vi "Get Command Field Width.vi"(8 "error in (no error)":errorcluster, 11 "RFFE Reg0Write Command in":refnum<class "RFFE Reg0Write Command.lvclass">) -> (0 "error out":errorcluster, 2 "Command Field Width":i32, 3 "RFFE Reg0Write Command out":refnum<class "RFFE Reg0Write Command.lvclass">)   [LabVIEW 2018, in "MIPI RFFE API.lvlib" / "RFFE Reg0Write Command.lvclass"]
uses:
  RFFE Reg0Write Command.lvclass
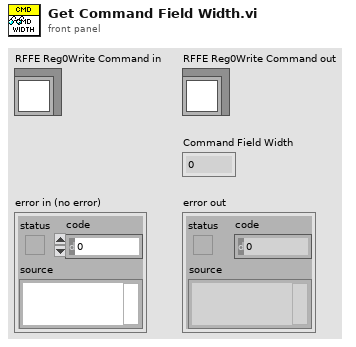
[diagram p1: front panel]
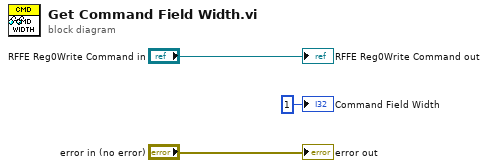
[diagram p0: block diagram]
diagram:
  "error out" <- "error in (no error)"
  "RFFE Reg0Write Command out" <- "RFFE Reg0Write Command in"
  "Command Field Width" <- 1 ("Command Field Width")
